vi "Progress Bar Initialization.vi"(1 "Array":dbl[][](array[numeric]), 2 "Trigger Snap or Scan?":bool, 3 "error in (no error)":errorcluster) -> (7 "Scan Progress":T1, 10 "error out":errorcluster)   [LabVIEW 2016]
uses:
  Controls/ScanParameters/Progress_Indicator.ctl
panel:
  # "of"
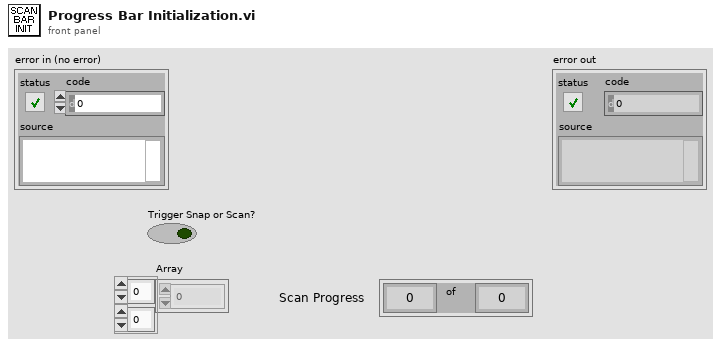
[diagram p1: front panel]
types:
  T1 = typedef "Progress_Indicator.ctl" = cluster{"Current Pnt Num":i32, "Total Num Pts":i32}
  T2 = typedef "Control 1" = cluster{"Current Pnt Num":i32, "Total Num Pts":i32}
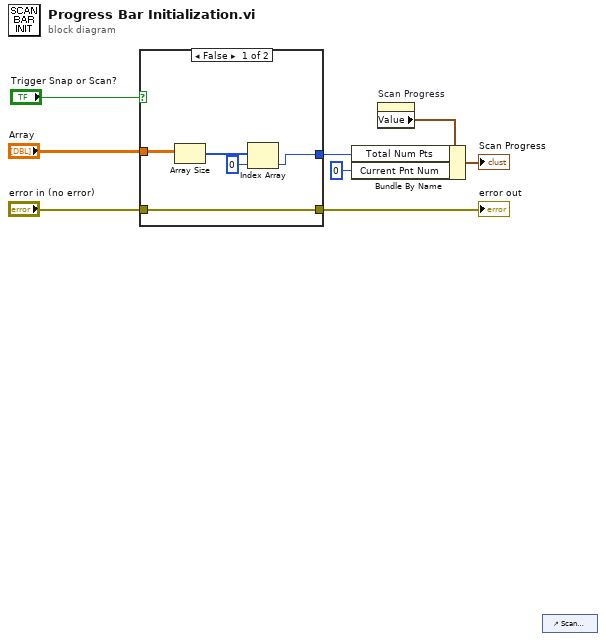
[diagram p0: block diagram]
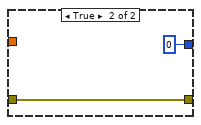
[diagram p2: hidden frame]
diagram:
  n1 = case shown="False" "Trigger Snap or Scan?" {
    tunnel: "Array" -> [w13 _]
    tunnel: "error in (no error)" -> [w9 w15]
    tunnel: [w9 w15] -> w6
    tunnel: [w10 0] -> w2
    frame False {
      n2 = Array Size(array=w13) -> (size(s)=w12:i32[])
      n3 = Index Array(array=w12, index=0) -> (element=w10:i32)
    }
    frame True {
    }
  }
  "error out" <- w6
  n4 = property on="Scan Progress" class="Clust (strict)"() -> ("Value"=w3:T2)  [unwired: 2 in, 2 out]
  n5 = Bundle By Name(cluster=w3, "Total Num Pts"=w2, "Current Pnt Num"=0) -> (→"Scan Progress":T2)
  n6 = control-ref of="Scan Progress"() -> ()  [unwired: 1 out]
